vi "Active.vi"(8 "error in (no error)":errorcluster, 11 "RToggleStream in":refnum<class "RToggleStream.lvclass">) -> (0 "error out":errorcluster, 2 "Active":bool, 3 "RToggleStream out":refnum<class "RToggleStream.lvclass">)   [LabVIEW 2020, in "obs-websocket.lvlib" / "RToggleStream.lvclass"]
uses:
  RToggleStream.lvclass
  RToggleStream.lvclass/RToggleStream.ctl
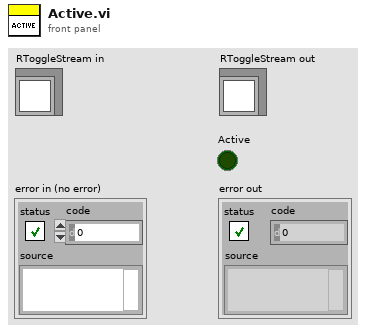
[diagram p1: front panel]
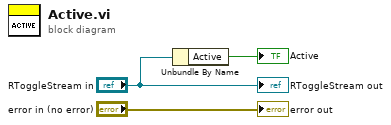
[diagram p0: block diagram]
diagram:
  n1 = Unbundle By Name("RToggleStream in") -> ("Active"=→"Active":bool)
  "error out" <- "error in (no error)"
  "RToggleStream out" <- "RToggleStream in"
